vi "Rename LVLIBs in LVPROJ XML File.vi"(7 "template base name":string, 8 "error in":errorcluster, 9 "CD name":string, 10 "relative path of LVLIB folders":path[](array[path]), 11 "custom device path":path) -> (0 "error out":errorcluster, 3 "custom device path out":path)   [LabVIEW 2020, in "Template Tool.lvlib"]
uses:
  Template Tool.lvlib
panel:
  out "number of replacements":i32[](array[numeric])
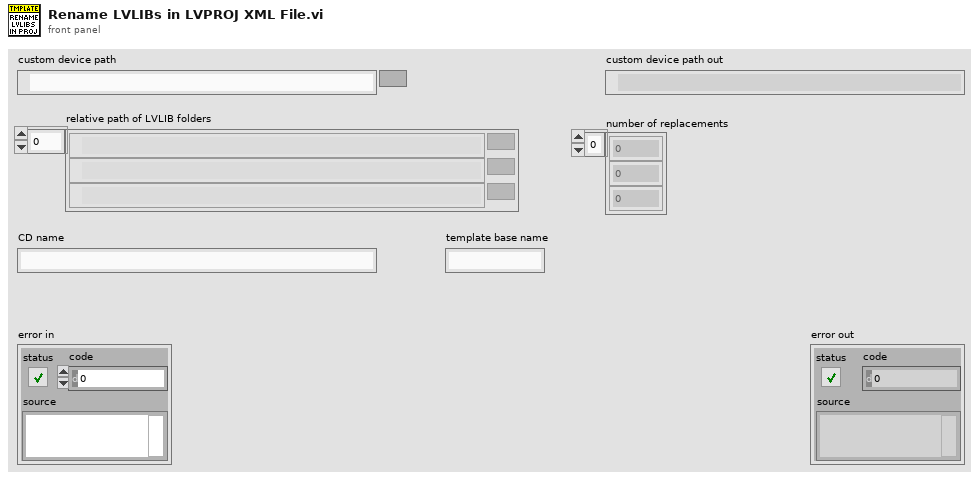
[diagram p1: front panel]
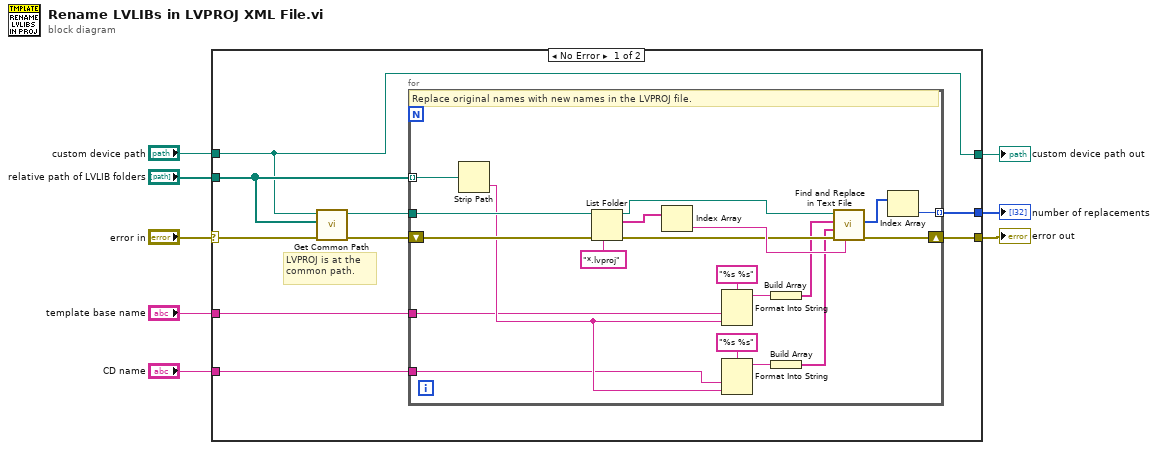
[diagram p0: block diagram]
diagram:
  n1 = case shown="No Error" "error in" {
    selector: "error in" -> [w15 w39]
    tunnel: "custom device path" -> [w12 w38]
    tunnel: [w17 w39] -> w7
    tunnel: [w12 w38] -> w6
    tunnel: "relative path of LVLIB folders" -> [w13 _]
    tunnel: [w16 _] -> w3
    tunnel: "CD name" -> [w10 _]
    tunnel: "template base name" -> [w9 _]
    frame No Error {
      # "LVPROJ is at the common path."
      n2 = call "Get Common Path.vi"("error in"=w15, "relative path of LVLIB folders"=w13, "custom device path"=w12) -> ("error out"=w14:errorcluster, "common path"=w11:path)  [unwired: 7 in]
      n3 = for {
        tunnel: w13 -> [w34] mode=indexing
        tunnel: [w20] -> w16 mode=indexing
        shift-right: [w30] -> w17
        shift-left: w14 -> [w37]
        tunnel: w11 -> [w26]
        tunnel: w10 -> [w19]
        tunnel: w9 -> [w18]
        # "Replace original names with new names in the LVPROJ file."
        n4 = Strip Path(path=w34) -> (name=w21:string)  [unwired: 1 out]
        n5 = List Folder(path=w26, pattern="*.lvproj", error in=w37) -> (path out=w33:path, filenames=w36:string[], error out=w31:errorcluster)  [unwired: 1 in, 1 out]
        n6 = Index Array(array=w36) -> (element=w32:string)  [unwired: 1 in]
        n7 = Format Into String(format string="%s %s", w18, w21) -> (resulting string=w24:string)  [unwired: 2 in, 1 out]
        n8 = Format Into String(format string="%s %s", w19, w21) -> (resulting string=w23:string)  [unwired: 2 in, 1 out]
        n9 = Build Array(w24) -> (w29:string[])
        n10 = Build Array(w23) -> (w28:string[])
        n11 = call "Find and Replace in Text File.vi"("file name"=w32, "error in"=w31, "replace array"=w28, "find array"=w29, "folder path"=w33) -> ("error out"=w30:errorcluster, "number of replacements"=w27:i32[])  [unwired: 5 in]
        n12 = Index Array(array=w27) -> (element=w20:i32)  [unwired: 1 in]
      }
    }
    frame Error {
    }
  }
  "error out" <- w7
  "custom device path out" <- w6
  "number of replacements" <- w3
